vi "DrawRectangle.vi"(0 "reference in":refnum<class "LcPictureBox.lvclass">, 1 "Rectangle":T3, 3 "Color(Black)":u32(colorbox), 4 "Alpha(100%)":dbl=100.0 min=0.0 max=100.0 format="%#_g%%", 5 "Error In":errorcluster, 7 "Fill(False)":bool, 8 "SmoothingMode(None)":T1, 9 "Pen(Width=1, Solid)":T2={"Width"=1, "Style"=enum."Solid"}) -> (14 "reference out":refnum<class "LcPictureBox.lvclass">, 19 "Error Out":errorcluster)   [LabVIEW 2020, in "LcPictureBox.lvclass"]
uses:
  LcPictureBox.lvclass
  System.Drawing
  Pen.ctl
  SmoothingMode.ctl
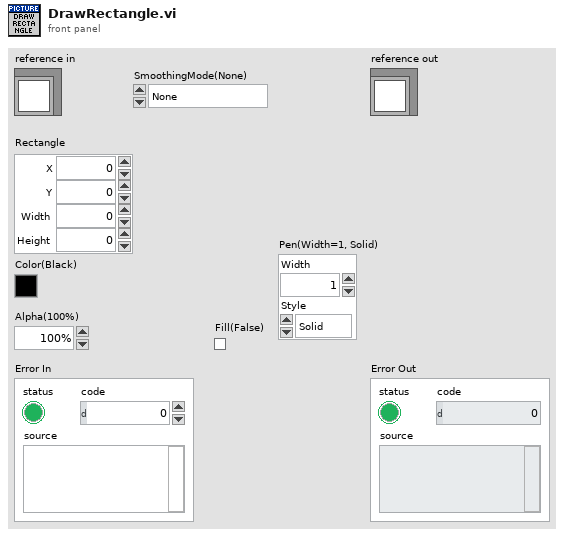
[diagram p1: front panel]
types:
  T1 = typedef "LcPictureBox.lvclass/SmoothingMode.ctl" = enum16{"None", "HighSpeed", "HighQuality", "AntiAlias"}
  T2 = typedef "LcPictureBox.lvclass/Pen.ctl" = cluster{"Width":u16, "Style":enum32{"Solid", "Dash", "Dot", "DashDot", "DashDotDot"}}
  T3 = cluster{"X":sgl, "Y":sgl, "Width":sgl, "Height":sgl}
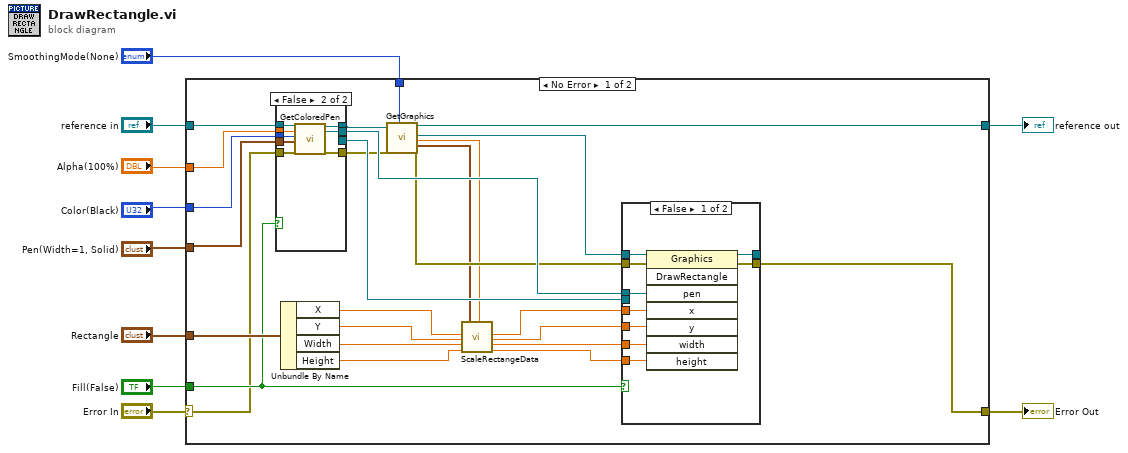
[diagram p0: block diagram]
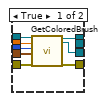
[diagram p2: hidden frame]
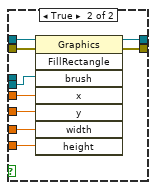
[diagram p3: hidden frame]
diagram:
  n1 = case shown="No Error" "Error In" {
    selector: "Error In" -> [w28 w72]
    tunnel: [w34 w72] -> w9
    tunnel: [w36 w71] -> w7
    tunnel: "reference in" -> [w33 w71]
    tunnel: "SmoothingMode(None)" -> [w21 _]
    tunnel: "Color(Black)" -> [w26 _]
    tunnel: "Alpha(100%)" -> [w27 _]
    tunnel: "Pen(Width=1, Solid)" -> [w25 _]
    tunnel: "Rectangle" -> [w35 _]
    tunnel: "Fill(False)" -> [w29 _]
    frame No Error {
      n2 = case shown="False" w29 {
        tunnel: [w44 w52] -> w32
        tunnel: w33 -> [w43 w51]
        tunnel: w28 -> [w42 w50]
        tunnel: [w41 w49] -> w24
        tunnel: w27 -> [w40 w48]
        tunnel: w26 -> [w39 w47]
        tunnel: w25 -> [w38 w46]
        tunnel: [_ w45] -> w31
        tunnel: [w37 _] -> w30
        frame True {
          n3 = call "GetColoredBrush.vi"("reference in"=w43, "Alpha(100%)"=w40, "Color(Black)"=w39, "Pen(Width=1, Solid)"=w38, "Error In"=w42) -> ("reference out"=w44:refnum<class "LcPictureBox.lvclass">, "SolidBrushRef"=w37:refnum<k24>, "Error Out"=w41:errorcluster)  [unwired: 12 in]
        }
        frame False {
          n4 = call "GetColoredPen.vi"("reference in"=w51, "Alpha(100%)"=w48, "Color(Black)"=w47, "Pen(Width=1, Solid)"=w46, "Error In"=w50) -> ("reference out"=w52:refnum<class "LcPictureBox.lvclass">, "PenRef"=w45:refnum<k24>, "Error Out"=w49:errorcluster)  [unwired: 12 in]
        }
      }
      n5 = Unbundle By Name(w35) -> ("X"=w18:sgl, "Y"=w17:sgl, "Width"=w16:sgl, "Height"=w15:sgl)
      n6 = call "GetGraphics.vi"("LcPictureBox in"=w32, "error in (no error)"=w24, "SmoothingMode"=w21) -> ("LcPictureBox out"=w36:refnum<class "LcPictureBox.lvclass">, "Graphics"=w22:refnum<k24>, "Scale"=w20:sgl, "Offset"=w19:cluster{"x":sgl, "y":sgl}, "error out"=w23:errorcluster)  [unwired: 12 in]
      n7 = call "ScaleRectangeData.vi"("X-In"=w18, "Y-In"=w17, "Width-In"=w16, "Height-In"=w15, "Offset(raw)"=w19, "Scale"=w20) -> ("X-Out"=w14:sgl, "Y-Out"=w13:sgl, "Width-Out"=w12:sgl, "Height-Out"=w11:sgl)  [unwired: 10 in]
      n8 = case shown="False" w29 {
        tunnel: w22 -> [w61 w70]
        tunnel: w23 -> [w60 w69]
        tunnel: [w59 w68] -> _
        tunnel: [w58 w67] -> w34
        tunnel: w14 -> [w57 w66]
        tunnel: w13 -> [w56 w65]
        tunnel: w12 -> [w55 w64]
        tunnel: w11 -> [w54 w63]
        tunnel: w31 -> [w53 _]
        tunnel: w30 -> [_ w62]
        frame False {
          n9 = invoke class="Graphics" method="DrawRectangle"(reference=w61, error in=w60, "pen"=w53, "x"=w57, "y"=w56, "width"=w55, "height"=w54) -> (reference out=w59:refnum<k24>, error out=w58:errorcluster)  [unwired: 1 in, 6 out]
        }
        frame True {
          n10 = invoke class="Graphics" method="FillRectangle"(reference=w70, error in=w69, "brush"=w62, "x"=w66, "y"=w65, "width"=w64, "height"=w63) -> (reference out=w68:refnum<k24>, error out=w67:errorcluster)  [unwired: 1 in, 6 out]
        }
      }
    }
    frame Error {
    }
  }
  "Error Out" <- w9
  "reference out" <- w7
